vi "Process_K7DRAMFIFO.vi"(9 "arbiter configuration":T1={"write grant time (clocks)"=100, "read grant time (clocks)"=100}, 11 "DRAM FIFO Ref In":refnum<class "K7 DRAM FIFO.lvclass">) -> ()   [LabVIEW 2015, in "K7 DRAM FIFO.lvclass"]
doc: "This VI manages the transfer of enqueued elements to and from the DRAM. This VI must execute in a SCTL that uses the DRAM Clock as a timing source.\n\n<B>Inputs</B>\n<B>DRAM FIFO Ref In</B> specifies the FIFO that the process manages.\n<B>write grant time (clocks)</B> specifies the number of consecutive writes to DRAM before switching back to reads.\n<B>read grant time (clocks)</B> specifies the number of consecutive reads from DRAM before switching back to writes\n\n<B>Detailed Help</B>\nThe DRAM FIFO Process must be placed within a SCTL that uses the \"DRAM Clock\" as a timing source.\n\nDRAM can not perform a read and write at the same time, thus performance is optimized by alternating between consecutive reads then consecutive writes."
uses:
  K7 DRAM FIFO.lvclass
  <vilib>/rvi/DataTransferAndStorage/Container/XNode/niFpgaContainer.xnode
  <instrlib>/_niInstr/Memory/v1/FPGA/Memory/Public/Read Request.ctl
  <instrlib>/_niInstr/Memory/v1/FPGA/Memory/niInstr Memory v1 FPGA.lvclass
  <instrlib>/_niInstr/Memory/v1/FPGA/Memory/Public/Write Data (With Byte Enables).ctl
  <instrlib>/_niInstr/Basic Elements/v1/FPGA/niInstr Basic Elements v1 FPGA.lvlib
  <instrlib>/_niInstr/Basic Elements/v1/FPGA/Private/Count Down U32.vi
  <vilib>/rvi/FIFO/Fifo_Resource/niFpgaFifoEmulationRefIn.vi
  <instrlib>/_niInstr/Memory/v1/FPGA/DRAM/niInstr Memory DRAM v1 FPGA.lvclass
  <instrlib>/_niInstr/Memory/v1/FPGA/DRAM/Public/Timeslot Arbiter Configuration.ctl
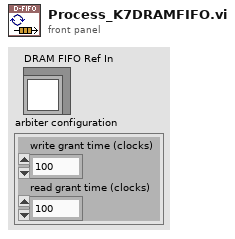
[diagram p1: front panel]
types:
  T1 = typedef "niInstr Memory DRAM v1 FPGA.lvclass/Timeslot Arbiter Configuration.ctl" = cluster{"write grant time (clocks)":u16, "read grant time (clocks)":u16}
  T2 = typedef "niInstr Memory v1 FPGA.lvclass/Write Data (With Byte Enables).ctl" = cluster{"address":u32, "data":bool[], "byte enables":bool[], "valid":bool}
  T3 = typedef "niInstr Memory v1 FPGA.lvclass/Read Request.ctl" = cluster{"address":u32, "valid":bool}
  T4 = typedef "Control 1.ctl" = dbl
  T5 = typedef "niInstr Memory v1 FPGA.lvclass/Retrieve Data.ctl" = cluster{"data":bool[], "valid":bool}
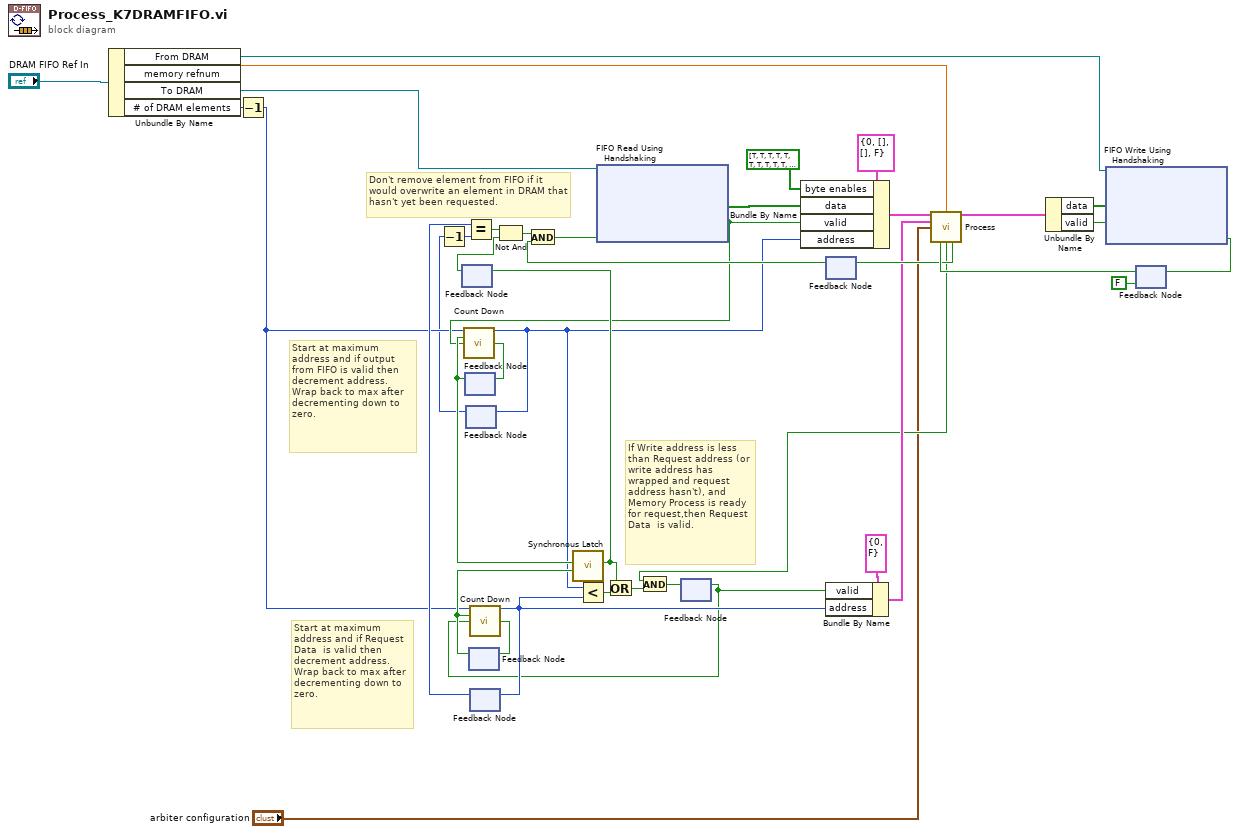
[diagram p0: block diagram]
diagram:
  # "If Write address is less than Request address (or write address has wrapped and request address hasn't), and Memory Process is ready for request,then Request Data  is valid."
  # "Start at maximum address and if Request Data  is valid then decrement address. Wrap back to max after decrementing down to zero."
  # "Start at maximum address and if output from FIFO is valid then decrement address. Wrap back to max after decrementing down to zero."
  # "Don't remove element from FIFO if it would overwrite an element in DRAM that hasn't yet been requested."
  n1 = Unbundle By Name("DRAM FIFO Ref In") -> ("From DRAM"=w5:refnum<k21>, "memory refnum"=w6:T4, "To DRAM"=w2:refnum<k21>, "# of DRAM elements"=w7:u32)
  n2 = Decrement(x=w7) -> (x-1=w10:u32)
  n3 = feedback #1() -> (w17:bool)  [unwired: 1 in]
  n4 = feedback #2() -> (w27:bool)  [unwired: 1 in]
  n5 = feedback #3() -> (w3:u32)  [unwired: 1 in]
  n6 = Decrement(x=w3) -> (x-1=w4:u32)
  n7 = feedback #4() -> (w28:bool)  [unwired: 1 in]
  n8 = feedback #5() -> (w14:u32)  [unwired: 1 in]
  n9 = Equal?(x=w14, y=w4) -> (x = y?=w19:bool)
  n10 = Not And(1:w17, 2:w19) -> (0:w22:bool)
  n11 = call <instrlib>:"Synchronous Latch.vi"("clear"=w28, "set"=w27) -> ("out"=w18:bool)  [unwired: 9 in]
  n12 = feedback-in #1(w18) -> ()
  n13 = feedback #6() -> (w11:bool)  [unwired: 1 in]
  n14 = call-poly <instrlib>:"Count Down.vi"("count in"=w10, "load"=w28, "decrement"=w11) -> ("count out"=w15:u32, "terminal count"=w29:bool)  [unwired: 11 in]
  n15 = feedback-in #4(w29) -> ()
  n16 = feedback-in #5(w15) -> ()
  n17 = feedback #7() -> (w21:bool)  [unwired: 1 in]
  n18 = And(x=w22, y=w21) -> (x .and. y?=w20:bool)
  n19 = xnode ("FIFO Read Using Handshaking")("Ready for Output"=w20, "FIFO In"=w2) -> ("Element"=w40:bool[], "Output Valid"=w12:bool)  [unwired: 1 out]
  n20 = call-poly <instrlib>:"Count Down.vi"("count in"=w10, "load"=w27, "decrement"=w12) -> ("count out"=w16:u32, "terminal count"=w30:bool)  [unwired: 11 in]
  n21 = feedback-in #2(w30) -> ()
  n22 = feedback-in #3(w16) -> ()
  n23 = Less?(x=w16, y=w15) -> (x < y?=w26:bool)
  n24 = Or(x=w18, y=w26) -> (x .or. y?=w25:bool)
  n25 = Bundle By Name(cluster=T2 {"address"=0, "data"=[], "byte enables"=[], "valid"=FALSE} ("write"), "byte enables"=bool[] [TRUE, TRUE, TRUE, TRUE, TRUE, TRUE, TRUE, TRUE, TRUE, TRUE, TRUE, TRUE, TRUE, TRUE, TRUE, TRUE, TRUE, TRUE, TRUE, TRUE, TRUE, TRUE, TRUE, TRUE, TRUE, TRUE, TRUE, TRUE, TRUE, TRUE, TRUE, TRUE, TRUE, TRUE, TRUE, TRUE, TRUE, TRUE, TRUE, TRUE, TRUE, TRUE, TRUE, TRUE, TRUE, TRUE, TRUE, TRUE, TRUE, TRUE, TRUE, TRUE, TRUE, TRUE, TRUE, TRUE, TRUE, TRUE, TRUE, TRUE, TRUE, TRUE, TRUE, TRUE], "data"=w40, "valid"=w12, "address"=w16) -> (w36:T2)
  n26 = Bundle By Name(cluster=T3 {"address"=0, "valid"=FALSE} ("request data"), "valid"=w11, "address"=w15) -> (w32:T3)
  n27 = feedback #8(FALSE ("Ready for Input")) -> (w41:bool)
  n28 = call-dynamic "Process.vi"("write"=w36, "memory"=w6, "request data"=w32, "arbiter configuration"="arbiter configuration", "ready for retrieve data (T)"=w41) -> ("retrieve data"=w37:T5, "ready for request data"=w23:bool, "ready for write"=w39:bool)  [unwired: 7 in, 1 out]
  n29 = And(x=w23, y=w25) -> (x .and. y?=w24:bool)
  n30 = feedback-in #6(w24) -> ()
  n31 = feedback-in #7(w39) -> ()
  n32 = Unbundle By Name(w37) -> ("data"=w9:bool[], "valid"=w13:bool)
  n33 = xnode ("FIFO Write Using Handshaking")("Element"=w9, "Input Valid"=w13, "FIFO In"=w5) -> ("Ready for Input"=w38:bool)  [unwired: 1 out]
  n34 = feedback-in #8(w38) -> ()
